vi "HTML_Title_Scraper.vi"() -> ()   [LabVIEW 2019]
uses:
  <vilib>/httpClient/LabVIEWHTTPClient.lvlib
panel:
  in  "url":string="https://www.pxl.be"
  out "<title> tag":string
  out "body":string
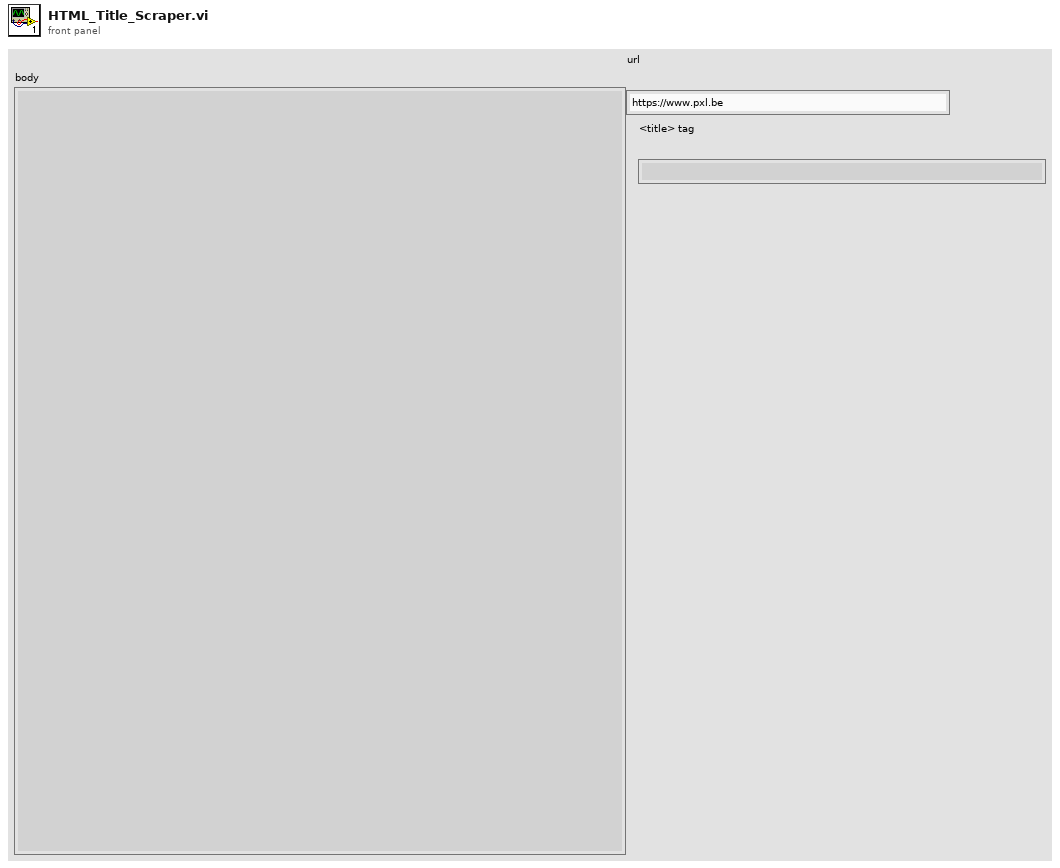
[diagram p1: front panel]
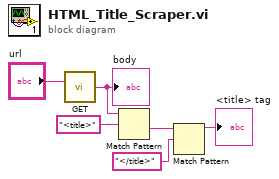
[diagram p0: block diagram]
diagram:
  n1 = call <vilib>:"GET.vi"("url"="url") -> ("body"=w4:string)  [unwired: 11 in, 3 out]
  "body" <- w4
  n2 = Match Pattern(string=w4, regular expression="<title>" ("format string")) -> (after substring=w3:string)  [unwired: 1 in, 3 out]
  n3 = Match Pattern(string=w3, regular expression="</title>" ("format string")) -> (before substring=→"<title> tag":string)  [unwired: 1 in, 3 out]
